vi "runtest run test core.vi"(6 "Test Execution Settings":T5={"Quick Mode (T)"=FALSE, "Seq Count"=0, "Step Info"="", "Instruments on Station"=[], "LANGUAGE"="English", "Files Found?"=FALSE, "Step Number"=1} {"Step Number" min=1 step=1}, 7 "Fields In":T1[](array[typedef]), 8 "error in (no error)":errorcluster, 9 "Parameters":string, 10 "Test Path (empty)":path, 11 "application reference (local)":refnum<vi>) -> (0 "error out":errorcluster, 3 "dup application reference":refnum<vi>, 4 "Test Output":T4, 5 "Fields Out":T1[](array[typedef]))   [LabVIEW 2011]
uses:
  tests/Test Execution Settings.ctl
  server/database/Stations/Instruments/Instrument Record.ctl
  tests/Test Output.ctl
  server/database/Fields/Field Record.ctl
  server/database/Fields/Field DataTypes.ctl
  server/database/Fields/Field NextItem.ctl
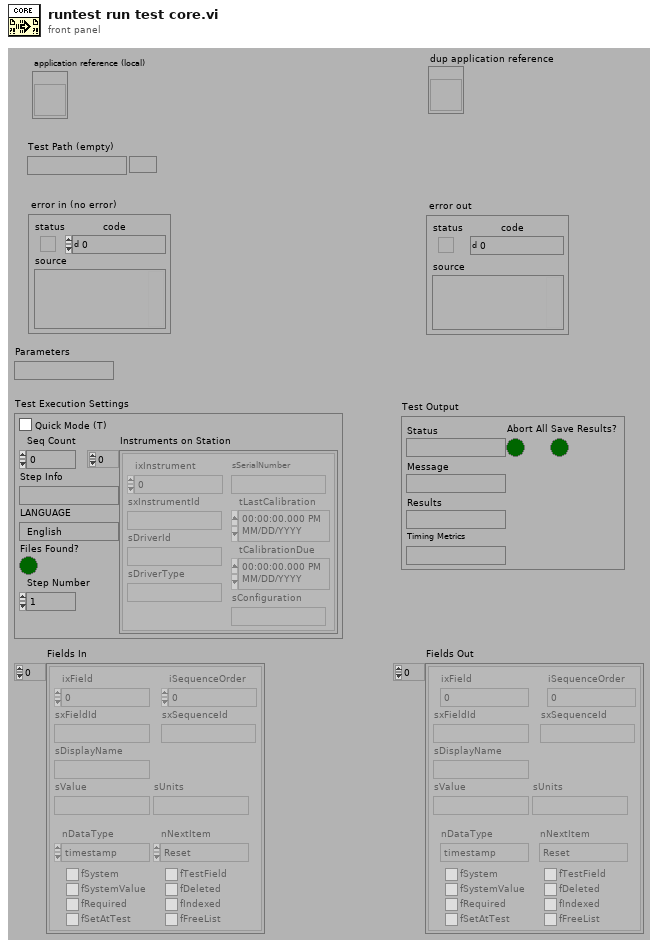
[diagram p1: front panel]
types:
  T1 = typedef "Field Record.ctl" = cluster{"ixField":i32, "iSequenceOrder":i32, "sxFieldId":string, "sxSequenceId":string, "sDisplayName":string, "sValue":string, "sUnits":string, "nDataType":T2, "nNextItem":T3, "fSystem":bool, "fSystemValue":bool, "fRequired":bool, "fSetAtTest":bool, "fTestField":bool, "fDeleted":bool, "fIndexed":bool, "fFreeList":bool}
  T2 = typedef "Field DataTypes.ctl" = enum32{"text", "numeric", "list", "timestamp", "boolean"}
  T3 = typedef "Field NextItem.ctl" = enum32{"Reset", "Retain", "Auto-Increment"}
  T4 = typedef "Test Output.ctl" = cluster{"Status":string, "Message":string, "Results":string, "Abort All":bool, "Save Results?":bool, "Timing Metrics":string}
  T5 = typedef "Test Execution Settings.ctl" = cluster{"Quick Mode (T)":bool, "Seq Count":i32, "Step Info":string, "Instruments on Station":T6[], "LANGUAGE":string, "Files Found?":bool, "Step Number":i32}
  T6 = typedef "Instrument Record.ctl" = cluster{"ixInstrument":i32, "sxInstrumentId":string, "sDriverId":string, "sDriverType":string, "sSerialNumber":string, "tLastCalibration":timestamp, "tCalibrationDue":timestamp, "sConfiguration":string}
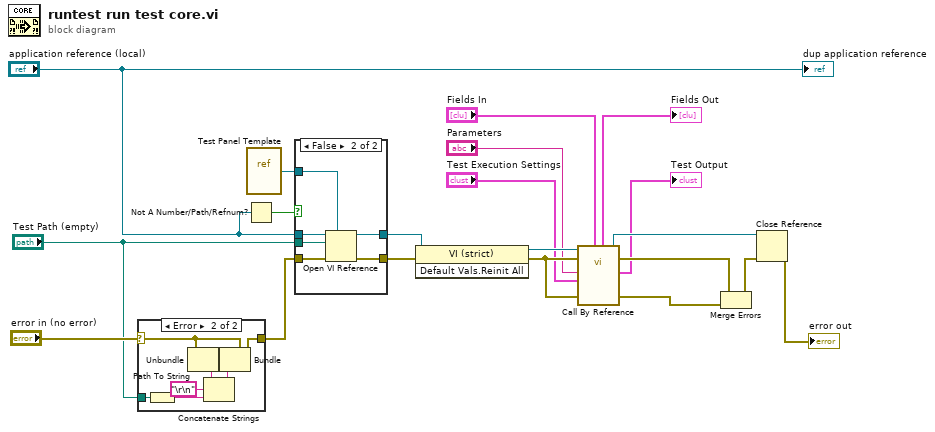
[diagram p0: block diagram]
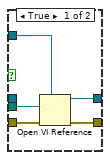
[diagram p2: hidden frame]
diagram:
  n1 = case shown="Error" "error in (no error)" {
    selector: "error in (no error)" -> [w21 w25]
    tunnel: "Test Path (empty)" -> [_ w27]
    tunnel: [w21 w22] -> w4
    frame No Error {
    }
    frame Error {
      n2 = Path To String(path=w27) -> (string=w26:string)
      n3 = Unbundle(w25) -> ("source"=w24:string)  [unwired: 2 out]
      n4 = Concatenate Strings(w24, "\r\n", w26) -> (w23:string)
      n5 = Bundle(cluster=w25, "source"=w23) -> (w22:errorcluster)  [unwired: 2 out]
    }
  }
  n6 = Not A Number/Path/Refnum?(number/path/refnum="application reference (local)") -> (NaN/Path/Refnum?=w1:bool)
  n7 = vi-ref "Test Panel Template.vi"() -> ("vi reference"=w20:refnum<vi>)
  n8 = case shown="False" w1 {
    tunnel: w20 -> [w33 w39]
    tunnel: [w32 w38] -> w15
    tunnel: [w31 w37] -> w14
    tunnel: "application reference (local)" -> [_ w34]
    tunnel: w4 -> [w30 w36]
    tunnel: "Test Path (empty)" -> [w29 w35]
    frame True {
      n9 = Open VI Reference(type specifier VI Refnum (for type only)=w33, vi path=w29, error in (no error)=w30) -> (vi reference=w31:refnum<vi>, error out=w32:errorcluster)  [unwired: 3 out]
    }
    frame False {
      n10 = Open VI Reference(type specifier VI Refnum (for type only)=w39, application reference (local)=w34, vi path=w35, error in (no error)=w36) -> (vi reference=w37:refnum<vi>, error out=w38:errorcluster)  [unwired: 2 out]
    }
  }
  n11 = invoke class="VI (strict)" method="Default Vals.Reinit All"(reference=w14, error in=w15) -> (reference out=w16:refnum<vi>, error out=w17:errorcluster)  [unwired: 1 in, 1 out]
  n12 = call-by-ref "?"(reference=w16, error in=w17, "Fields In"="Fields In", 8:"error in (no error)"=w17, "Test Execution Settings"="Test Execution Settings", "Parameters"="Parameters") -> (reference out=w12:refnum<vi>, error out=w19:errorcluster, 0:"error out"=w18:errorcluster, "Test Output"=→"Test Output":T4, "Fields Out"=→"Fields Out":T1[])  [unwired: 5 in]
  n13 = Merge Errors(w19, w18) -> (w13:errorcluster)
  n14 = Close Reference(reference=w12, error in (no error)=w13) -> (error out=→"error out":errorcluster)
  "dup application reference" <- "application reference (local)"
